vi "sftp_stat.vi"() -> ()   [LabVIEW 2017]
doc: "Illustrates how to read and write file information by path."
uses:
  libssh2/libssh2_session_handshake_tcp.vi
  libssh2/libssh2_init_default.vi
  libssh2/libssh2_session_init_ex.vi
  <vilib>/Utility/tcp.llb/TCP Get Raw Net Object.vi
  libssh2/libssh2_session_handshake_socket.vi
  libssh2/libssh2_userauth_password_ex.vi
  libssh2/libssh2_sftp_stat_ex.vi
  libssh2/libssh2.lvlib
panel:
  out "original mtime":timestamp
  out "new mtime":timestamp
  in  "file":string="/"
  out "error out":errorcluster
  in  "password":string
  in  "username":string
  in  "hostname":string
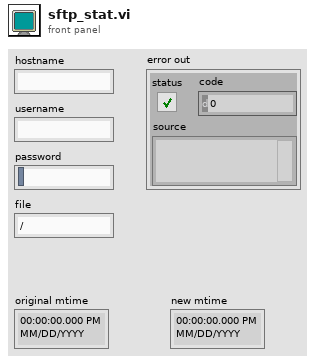
[diagram p1: front panel]
types:
  T1 = typedef "libssh2.lvlib/Session Refnum.ctl" = refnum<k1>
  T2 = typedef "libssh2.lvlib/SFTP Refnum.ctl" = refnum<k1>
  T3 = typedef "libssh2.lvlib/libssh2_sftp_attributes.ctl" = cluster{"flags":u32, "filesize":u64, "uid":u32, "gid":u32, "permissions":u32, "atime":u32, "mtime":u32}
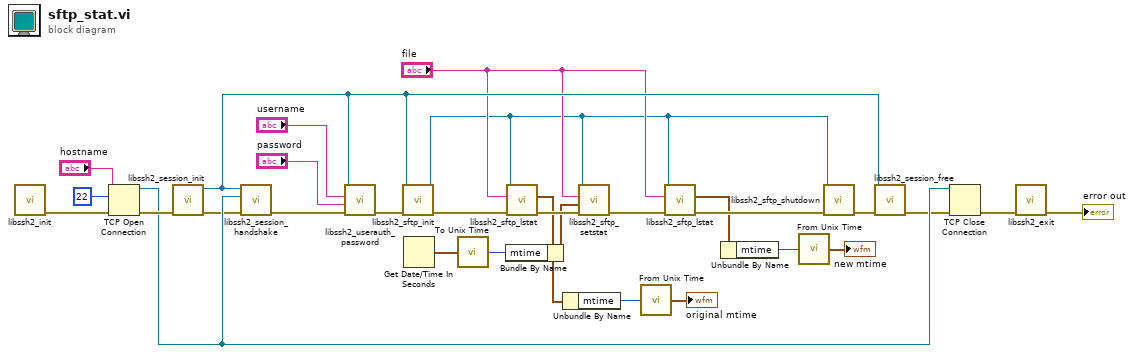
[diagram p0: block diagram]
diagram:
  n1 = call-poly "libssh2_init.vi"() -> ("error out"=w29:errorcluster)  [unwired: 11 in]
  n2 = TCP Open Connection(address="hostname", remote port or service name=u16 22, error in (no error)=w29) -> (connection ID=w27:refnum<k5>, error out=w28:errorcluster)  [unwired: 2 in]
  n3 = call "libssh2_session_init.vi"("error in (no error)"=w28) -> ("error out"=w26:errorcluster, "session"=w19:T1)  [unwired: 9 in]
  n4 = call-poly "libssh2_session_handshake.vi"("error in (no error)"=w26, "tcp connection"=w27, "session"=w19) -> ("error out"=w30:errorcluster)  [unwired: 8 in]
  n5 = call "libssh2_userauth_password.vi"("error in (no error)"=w30, "password"="password", "username"="username", "session"=w19) -> ("error out"=w23:errorcluster)  [unwired: 7 in]
  n6 = call "libssh2_sftp_init.vi"("error in (no error)"=w23, "session"=w19) -> ("error out"=w4:errorcluster, "sftp"=w1:T2)  [unwired: 8 in]
  n7 = Get Date/Time In Seconds() -> (seconds since 1Jan1904=w7:timestamp)
  n8 = call "To Unix Time.vi"("timestamp"=w7) -> ("unix time"=w8:u32)  [unwired: 1 in]
  n9 = call "libssh2_sftp_lstat.vi"("error in (no error)"=w4, "path"="file", "sftp"=w1) -> ("error out"=w15:errorcluster, "attributes"=w3:T3)  [unwired: 7 in]
  n10 = Bundle By Name(cluster=w3, "mtime"=w8) -> (w9:T3)
  n11 = Unbundle By Name(w3) -> ("mtime"=w5:u32)
  n12 = call "libssh2_sftp_setstat.vi"("error in (no error)"=w15, "attributes in"=w9, "path"="file", "sftp"=w1) -> ("error out"=w12:errorcluster)  [unwired: 7 in]
  n13 = call "From Unix Time.vi"("unix time"=w5) -> ("timestamp"=→"original mtime":timestamp)  [unwired: 1 in]
  n14 = call "libssh2_sftp_lstat.vi"("error in (no error)"=w12, "path"="file", "sftp"=w1) -> ("error out"=w11:errorcluster, "attributes"=w10:T3)  [unwired: 7 in]
  n15 = Unbundle By Name(w10) -> ("mtime"=w14:u32)
  n16 = call "From Unix Time.vi"("unix time"=w14) -> ("timestamp"=→"new mtime":timestamp)  [unwired: 1 in]
  n17 = call "libssh2_sftp_shutdown.vi"("error in (no error)"=w11, "sftp"=w1) -> ("error out"=w16:errorcluster)  [unwired: 9 in]
  n18 = call "libssh2_session_free.vi"("error in (no error)"=w16, "session"=w19) -> ("error out"=w18:errorcluster)  [unwired: 9 in]
  n19 = TCP Close Connection(connection ID=w27, error in (no error)=w18) -> (error out=w17:errorcluster)  [unwired: 1 in, 1 out]
  n20 = call "libssh2_exit.vi"("error in (no error)"=w17) -> ("error out"=→"error out":errorcluster)  [unwired: 10 in]
